vi "Read Setpoint Enable.vi"(8 "error in (no error)":errorcluster, 11 "VISA resource name":refnum<visa-resource-name>) -> (0 "error out":errorcluster, 1 "Setpoint Status":i16, 3 "VISA resource name out":refnum<visa-resource-name>)   [LabVIEW 2010, in "Temptronic TP04300.lvlib"]
doc: "This VI reads <b>Setpoint Enable</b>.\n\nValid range: 0 - Setpoint Disabled\n 1 - Setpoint Enabled"
uses:
  Temptronic TP04300.lvlib
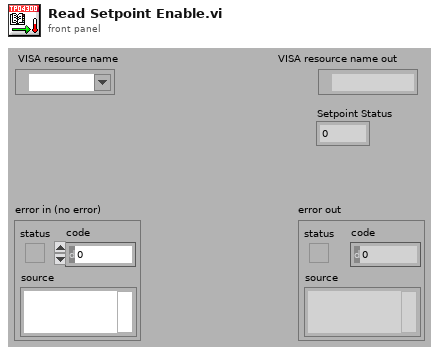
[diagram p1: front panel]
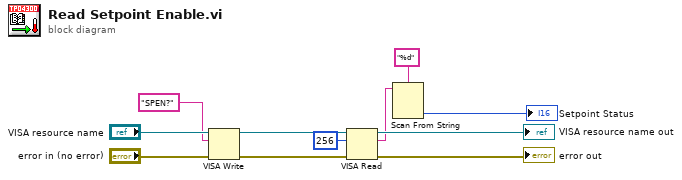
[diagram p0: block diagram]
diagram:
  n1 = VISA Write(VISA resource name="VISA resource name", write buffer="SPEN?" ("format string"), error in (no error)="error in (no error)") -> (VISA resource name out=w6:refnum<visa-resource-name>, error out=w9:errorcluster)  [unwired: 1 out]
  n2 = VISA Read(VISA resource name=w6, byte count=u32 256, error in (no error)=w9) -> (VISA resource name out=→"VISA resource name out":refnum<visa-resource-name>, read buffer=w4:string, error out=→"error out":errorcluster)  [unwired: 1 out]
  n3 = Scan From String(format string="%d", input string=w4) -> (output 1=→"Setpoint Status":i16)  [unwired: 3 in, 3 out]
